vi "hw4-3 topVI.vi"() -> ()   [LabVIEW 2014]
panel:
  out "samples per acquisition 2":dbl=10000.0
  out "sampling rate (samples/sec) 2":dbl=1000.0
  out "acquire":bool
  out "config":bool
  out "correct":bool
  in  "stop":bool
  in  "Menu cluster":cluster{bool, bool, bool}
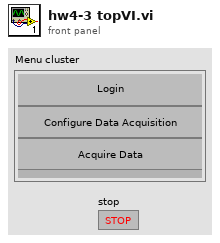
[diagram p1: front panel]
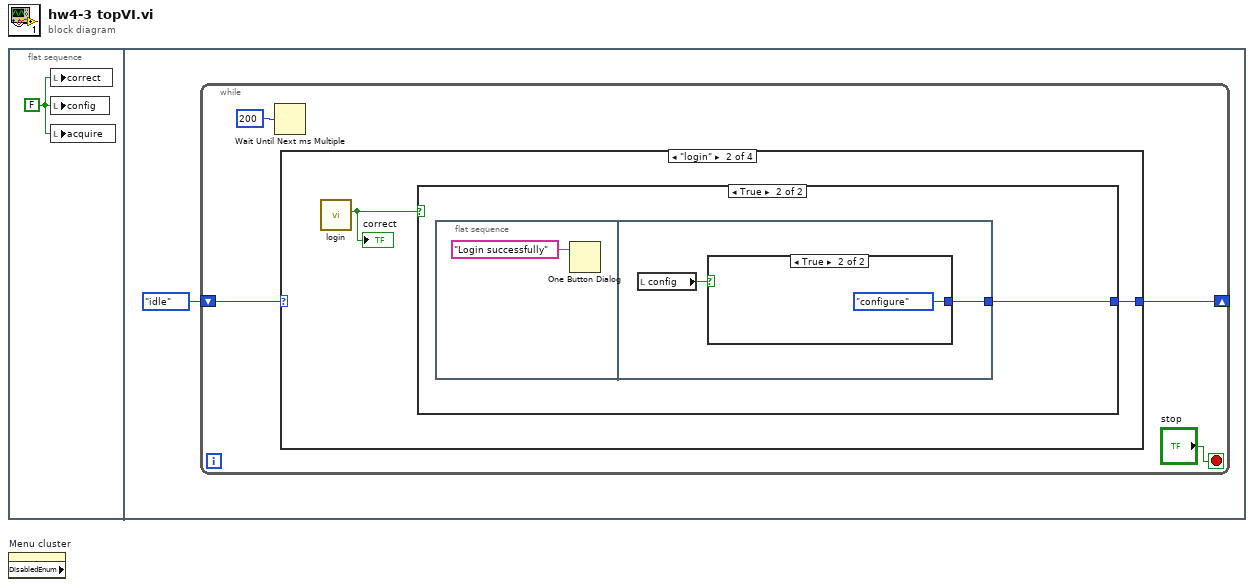
[diagram p0: block diagram]
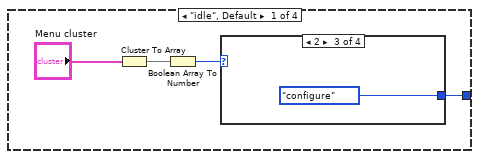
[diagram p2: hidden frame]
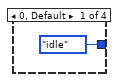
[diagram p3: hidden frame]
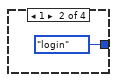
[diagram p4: hidden frame]
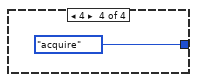
[diagram p5: hidden frame]
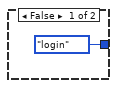
[diagram p6: hidden frame]
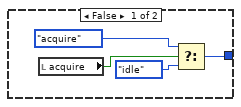
[diagram p7: hidden frame]
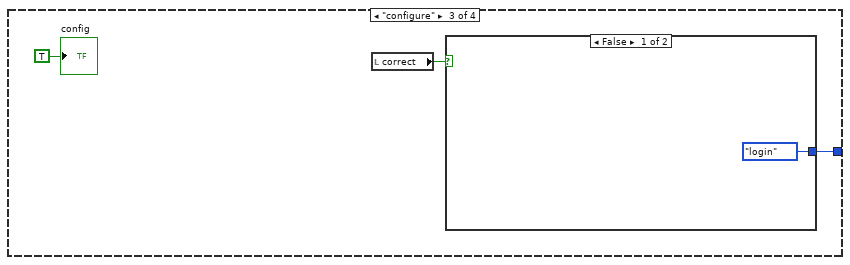
[diagram p8: hidden frame]
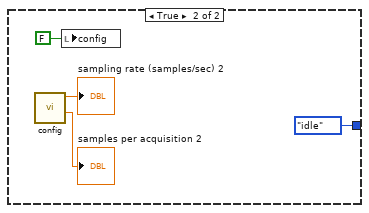
[diagram p9: hidden frame]
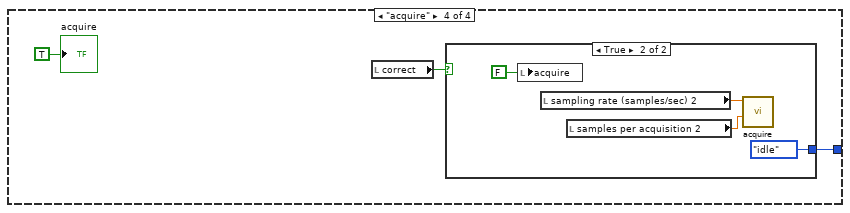
[diagram p10: hidden frame]
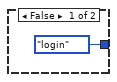
[diagram p11: hidden frame]
diagram:
  n1 = flat-sequence {
    frame #0 {
      w1 = FALSE
      n2 = local write "correct"(w1) -> ()
      n3 = local write "config"(w1) -> ()
      n4 = local write "acquire"(w1) -> ()
    }
    frame #1 {
      n5 = while {
        shift-right: [w4] -> _
        shift-left: enum16{"idle", "login", "configure", "acquire"}."idle" -> [w5]
        stop <- "stop" stop-if-true
        n6 = Wait Until Next ms Multiple(millisecond multiple=u32 200) -> ()  [unwired: 1 out]
        n7 = case shown="\"login\"" w5 {
          tunnel: [w7 w15 w28 w36] -> w4
          frame "idle", Default {
            n8 = Cluster To Array(cluster="Menu cluster") -> (array=w9:bool[])
            n9 = Boolean Array To Number(Boolean array=w9) -> (number=w8:u32)
            n10 = case shown="2" w8 {
              tunnel: [enum16{"idle", "login", "configure", "acquire"}."idle" enum16{"idle", "login", "configure", "acquire"}."login" enum16{"idle", "login", "configure", "acquire"}."configure" enum16{"idle", "login", "configure", "acquire"}."acquire"] -> w7
              frame 0, Default {
              }
              frame 1 {
              }
              frame 2 {
              }
              frame 4 {
              }
            }
          }
          frame "login" {
            n11 = call "login.vi"() -> ("correct"=w16:bool)  [unwired: 11 in]
            "correct" <- w16
            n12 = case shown="True" w16 {
              tunnel: [enum16{"idle", "login", "configure", "acquire"}."login" w18] -> w15
              frame False {
              }
              frame True {
                n13 = flat-sequence {
                  tunnel: [w20] -> w18
                  frame #0 {
                    n14 = One Button Dialog(message="Login successfully") -> ()  [unwired: 1 in, 1 out]
                  }
                  frame #1 {
                    n15 = local read "config"() -> (w21:bool)
                    n16 = case shown="True" w21 {
                      tunnel: [w24 enum16{"idle", "login", "configure", "acquire"}."configure"] -> w20
                      frame False {
                        n17 = local read "acquire"() -> (w25:bool)
                        n18 = Select(t=enum16{"idle", "login", "configure", "acquire"}."acquire", s=w25, f=enum16{"idle", "login", "configure", "acquire"}."idle") -> (s? t:f=w24:enum16{"idle", "login", "configure", "acquire"})
                      }
                      frame True {
                      }
                    }
                  }
                }
              }
            }
          }
          frame "configure" {
            n19 = local read "correct"() -> (w29:bool)
            n20 = case shown="False" w29 {
              tunnel: [enum16{"idle", "login", "configure", "acquire"}."login" enum16{"idle", "login", "configure", "acquire"}."idle"] -> w28
              frame False {
              }
              frame True {
                n21 = call "config.vi"() -> ("samples per acquisition 2"=→"samples per acquisition 2":dbl, "sampling rate (samples/sec) 2"=→"sampling rate (samples/sec) 2":dbl)  [unwired: 10 in]
                n22 = local write "config"(FALSE) -> ()
              }
            }
            "config" <- TRUE
          }
          frame "acquire" {
            n23 = local read "correct"() -> (w37:bool)
            n24 = case shown="True" w37 {
              tunnel: [enum16{"idle", "login", "configure", "acquire"}."login" enum16{"idle", "login", "configure", "acquire"}."idle"] -> w36
              frame False {
              }
              frame True {
                n25 = local write "acquire"(FALSE) -> ()
                n26 = local read "sampling rate (samples/sec) 2"() -> (w39:dbl)
                n27 = local read "samples per acquisition 2"() -> (w40:dbl)
                n28 = call "acquire.vi"("Samples per acquisition"=w40, "Sampling rate(samples/sec)"=w39) -> ()  [unwired: 10 in]
              }
            }
            "acquire" <- TRUE
          }
        }
      }
    }
  }
  n29 = property on="Menu cluster" class="Clust" props=["DisabledEnum"]() -> ()  [unwired: 2 in, 3 out]
